vi "Initialize.vi"(8 "error in (no error)":errorcluster, 11 "No Galvos in":refnum<class "No Galvos.lvclass">) -> (0 "error out":errorcluster, 3 "No Galvos out":refnum<class "No Galvos.lvclass">)   [LabVIEW 2015, in "No Galvos.lvclass"]
uses:
  No Galvos.lvclass
  Galvo.lvclass
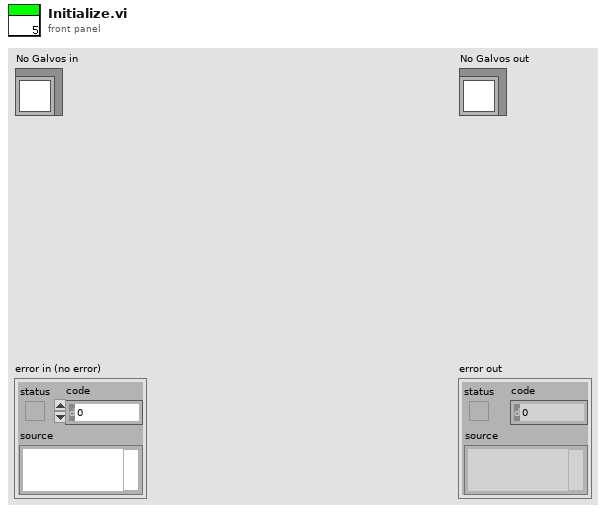
[diagram p1: front panel]
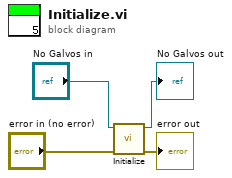
[diagram p0: block diagram]
diagram:
  n1 = call-parent "Initialize.vi"("error in (no error)"="error in (no error)", "Galvo in"="No Galvos in") -> ("error out"=→"error out":errorcluster, "Galvo out"=→"No Galvos out":refnum<class "No Galvos.lvclass">)  [unwired: 8 in]
